vi "Set Object Pointer.vi"(10 "Object Pointer":i64, 11 "Tree in":refnum<class "Tree.lvclass">) -> (3 "Tree out":refnum<class "Tree.lvclass">)   [LabVIEW 2012, in "MDSplus.lvlib" / "Tree.lvclass"]
uses:
  <vilib>/MDSplus/Classes/Tree_Class/Tree.lvclass
  <vilib>/MDSplus/Classes/Tree_Class/Tree.lvclass/Tree.ctl
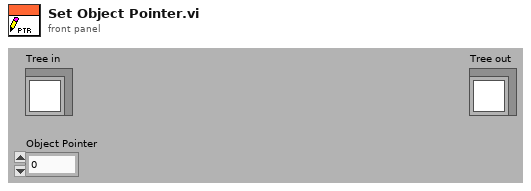
[diagram p1: front panel]
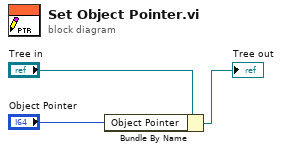
[diagram p0: block diagram]
diagram:
  n1 = Bundle By Name(cluster="Tree in", "Object Pointer"="Object Pointer") -> (→"Tree out":refnum<class "Tree.lvclass">)
